vi "Configure.vi"(8 "Error In":errorcluster, 11 "Configuration":T1) -> (0 "Error Out":errorcluster)   [LabVIEW 2014, in "LV-Logger.lvlib"]
uses:
  LV-Logger.lvlib
  Controls/Configuration.ctl
  Controls/Level.ctl
  Private/_File Manager Action.ctl
  Private/_Logger Action.ctl
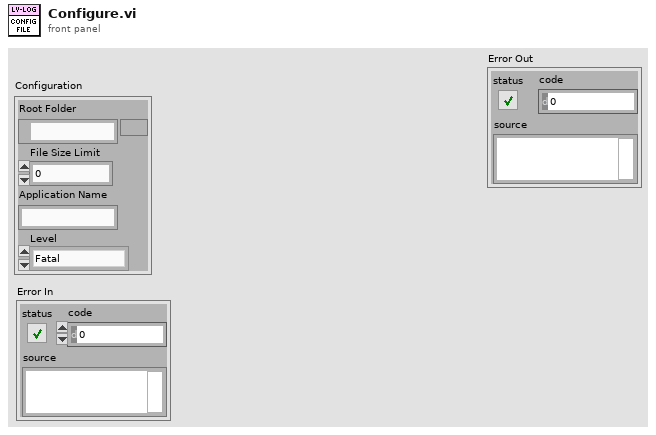
[diagram p1: front panel]
types:
  T1 = typedef "LV-Logger.lvlib/Configuration.ctl" = cluster{"Root Folder":path, "File Size Limit":i64, "Application Name":string, "Level":T2}
  T2 = typedef "LV-Logger.lvlib/Level.ctl" = enum16{"Fatal", "Error", "Warn", "Info", "Debug", "Trace"}
  T3 = typedef "LV-Logger.lvlib/_Logger Action.ctl" = enum16{"Initialize", "Register", "Log", "Unregister", "Set Level", "Shutdown"}
  T4 = typedef "LV-Logger.lvlib/_File Manager Action.ctl" = enum16{"Initialize", "Set File Size Limit", "Set Root Folder", "Set Application Name", "Start", "Write", "Stop", "Shutdown"}
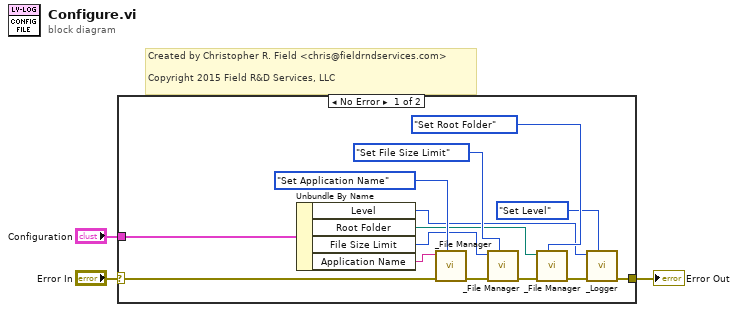
[diagram p0: block diagram]
diagram:
  # "Created by Christopher R. Field <chris@fieldrndservices.com>\n\nCopyright 2015 Field R&D Services, LLC"
  n1 = case shown="No Error" "Error In" {
    selector: "Error In" -> [w17 w18]
    tunnel: "Configuration" -> [w16 _]
    tunnel: [w6 w18] -> w1
    frame No Error {
      n2 = Unbundle By Name(w16) -> ("Level"=w5:T2, "Root Folder"=w8:path, "File Size Limit"=w11:i64, "Application Name"=w14:string)
      n3 = call "_File Manager.vi"("Action"=_File_Manager_Action."Set Application Name", "Error In"=w17, "Set Value"=w14) -> ("Error Out"=w13:errorcluster)  [unwired: 8 in]
      n4 = call "_File Manager.vi"("Action"=_File_Manager_Action."Set File Size Limit", "Error In"=w13, "Set Value"=w11) -> ("Error Out"=w10:errorcluster)  [unwired: 8 in]
      n5 = call "_File Manager.vi"("Action"=_File_Manager_Action."Set Root Folder", "Error In"=w10, "Set Value"=w8) -> ("Error Out"=w7:errorcluster)  [unwired: 8 in]
      n6 = call "_Logger.vi"("Action"=_Logger_Action."Set Level", "Error In"=w7, "Value In"=w5) -> ("Error Out"=w6:errorcluster)  [unwired: 8 in]
    }
    frame Error {
    }
  }
  "Error Out" <- w1
